vi "sym2w2.vi"(1 "Bits-per-Symbol":i32, 2 "Word-to-Symbol Map 2":cdb[](array[numeric]), 3 "Number of Subcarriers":i32, 4 "Parallel Symbol input":cdb[](array[numeric])) -> (0 "Parallel Word Output":bool[][](array[boolean]))   [LabVIEW 2013]
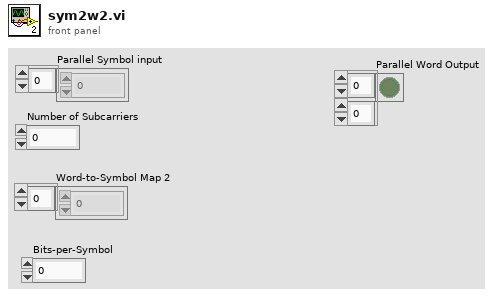
[diagram p1: front panel]
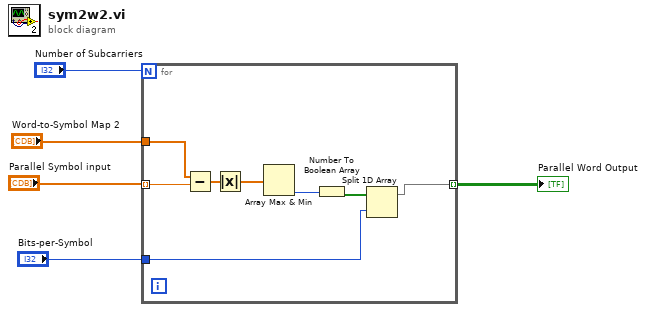
[diagram p0: block diagram]
diagram:
  n1 = for {
    N: "Number of Subcarriers" -> [_]
    tunnel: "Bits-per-Symbol" -> [w13]
    tunnel: [w10] -> w3 mode=indexing
    tunnel: "Word-to-Symbol Map 2" -> [w9]
    tunnel: "Parallel Symbol input" -> [w6] mode=indexing
    n2 = Subtract(x=w9, y=w6) -> (x-y=w8:cdb[])
    n3 = Absolute Value(x=w8) -> (abs(x)=w7:dbl[])
    n4 = Array Max & Min(array=w7) -> (min index (indices)=w12:i32)  [unwired: 3 out]
    n5 = Number To Boolean Array(number=w12) -> (Boolean array=w11:bool[])
    n6 = Split 1D Array(array=w11, index=w13) -> (first subarray=w10:bool[])  [unwired: 1 out]
  }
  "Parallel Word Output" <- w3
